vi "2.vi"(10 "FPGAReference":refnum<k20>, 11 "HealthAndStatusControlFIFO in":refnum<class "HealthAndStatusControlFIFO.lvclass">) -> (3 "HealthAndStatusControlFIFO out":refnum<class "HealthAndStatusControlFIFO.lvclass">)   [LabVIEW 2016]
uses:
  HealthAndStatusControlFIFO.lvclass
  D:/Code/ts_M1M3Support/Common_RT_FPGA/IWriteU64FIFO/IWriteU64FIFO.lvclass
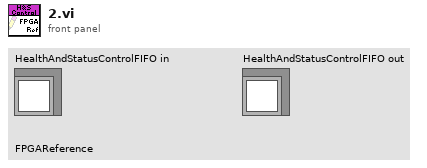
[diagram p1: front panel]
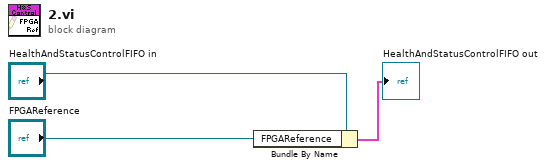
[diagram p0: block diagram]
diagram:
  n1 = Bundle By Name(cluster="HealthAndStatusControlFIFO in", "FPGAReference"="FPGAReference") -> (→"HealthAndStatusControlFIFO out":cluster{})
